vi "실습 2-2 복합연산.vi"() -> ()   [LabVIEW 2014]
panel:
  out "A 7":dbl
  in  "A 6":dbl
  in  "A 5":dbl
  in  "A 4":dbl
  in  "A 3":dbl
  in  "A 2":dbl
  in  "A":dbl
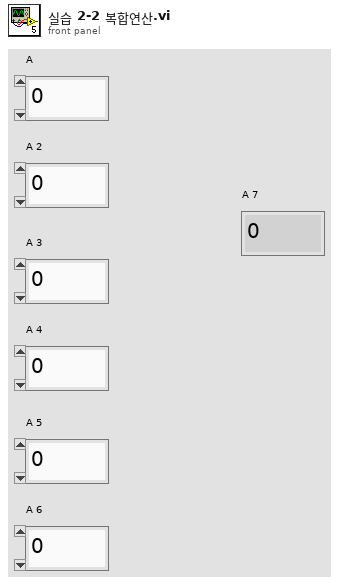
[diagram p1: front panel]
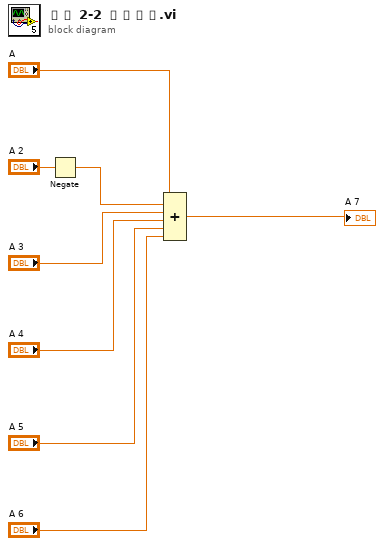
[diagram p0: block diagram]
diagram:
  n1 = Negate(x="A 2") -> (-x=w1:dbl)
  n2 = Compound Arithmetic op=ADD("A", w1, "A 3", "A 4", "A 5", "A 6") -> (→"A 7":dbl)
